vi "Rename Logs.vi"(8 "error in (no error)":errorcluster, 11 "Trace Controller in":refnum<class "Trace Controller.lvclass">) -> (0 "error out":errorcluster, 3 "Trace Controller out":refnum<class "Trace Controller.lvclass">)   [LabVIEW 2014, in "Robot Actor Framework.lvlib" / "Trace.lvlib" / "Trace Controller.lvclass"]
uses:
  Trace Controller.lvclass
  Trace Controller.lvclass/Trace Controller.ctl
panel:
  in  "Logs to Keep":i32=5
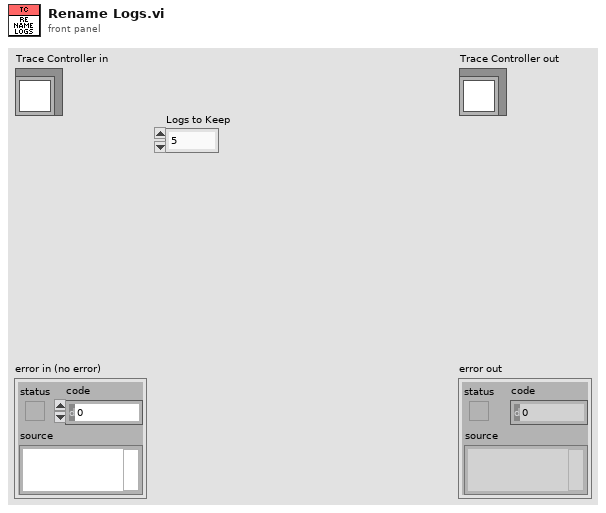
[diagram p1: front panel]
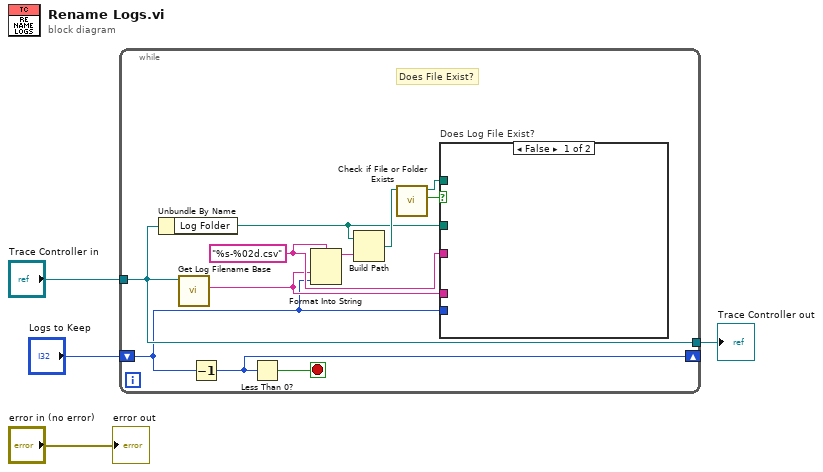
[diagram p0: block diagram]
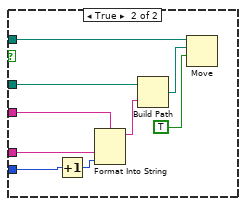
[diagram p2: hidden frame]
diagram:
  n1 = while {
    tunnel: "Trace Controller in" -> [w7]
    shift-right: [w9] -> _
    shift-left: "Logs to Keep" -> [w5]
    tunnel: [w7] -> w2
    stop <- w8 stop-if-true
    w11 = "%s-%02d.csv" ("format string")
    # "Does File Exist?"
    n2 = Unbundle By Name(w7) -> ("Log Folder"=w10:path)
    n3 = call-dynamic "Get Log Filename Base.vi"("Trace Controller in"=w7) -> ("Log Filename Base"=w6:string)  [unwired: 8 in, 2 out]
    n4 = Decrement(x=w5) -> (x-1=w9:i32)
    n5 = Less Than 0?(x=w9) -> (x < 0?=w8:bool)
    n6 = Format Into String(format string=w11, w6, w5) -> (resulting string=w15:string)  [unwired: 2 in, 1 out]
    n7 = Build Path(base path=w10, name or relative path=w15) -> (appended path=w14:path)
    n8 = call <vilib>:"Check if File or Folder Exists.vi"("path"=w14) -> ("file or folder exists?"=w13:bool, "dup path"=w12:path)  [unwired: 8 in, 1 out]
    n9 = case "Does Log File Exist?" shown="False" w13 {
      tunnel: w12 -> [_ w24]
      tunnel: w11 -> [_ w23]
      tunnel: w5 -> [_ w22]
      tunnel: w10 -> [_ w18]
      tunnel: w6 -> [_ w16]
      frame False {
      }
      frame True {
        n10 = Increment(x=w22) -> (x+1=w17:i32)
        n11 = Format Into String(format string=w23, w16, w17) -> (resulting string=w20:string)  [unwired: 2 in, 1 out]
        n12 = Build Path(base path=w18, name or relative path=w20) -> (appended path=w21:path)
        n13 = Move(source path=w24, 9:TRUE ("overwrite (F)"), 10:w21) -> ()  [unwired: 2 in, 3 out]
      }
    }
  }
  "Trace Controller out" <- w2
  "error out" <- "error in (no error)"
